vi "Pneumatic Control Loop.vi"(11 "Cluster in":T1) -> ()   [LabVIEW 2015]
uses:
  Support Code/Solenoid Control Loop.ctl
  Support Code/Pneumatics Command.ctl
  Support Code/Pneumatics Position.ctl
  <vilib>/Rock Robotics/WPI/Solenoid/WPI_SolenoidDevRef.ctl
  <vilib>/Rock Robotics/WPI/Solenoid/WPI_SolenoidChannel.ctl
  <vilib>/Rock Robotics/WPI/Solenoid/WPI_SolenoidValue.ctl
  <vilib>/Rock Robotics/WPI/Solenoid/WPI_SolenoidSetEnum.vi
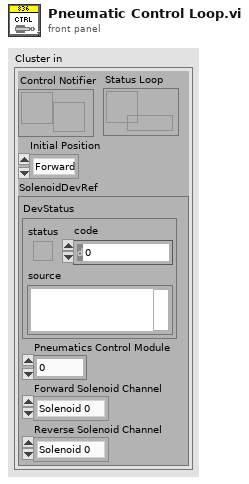
[diagram p1: front panel]
types:
  T1 = typedef "Solenoid Control Loop.ctl" = cluster{"Control Notifier":refnum<notifier>, "Initial Position":T2, "SolenoidDevRef":T3, "Status Loop":refnum<k33>}
  T2 = typedef "Pneumatics Position.ctl" = enum16{"Forward", "Reverse"}
  T3 = typedef "WPI_SolenoidDevRef.ctl" = cluster{"DevStatus":errorcluster, "Pneumatics Control Module":u8, "Forward Solenoid Channel":T4, "Reverse Solenoid Channel":T4}
  T4 = typedef "WPI_SolenoidChannel.ctl" = enum8{"Solenoid 0", "Solenoid 1", "Solenoid 2", "Solenoid 3", "Solenoid 4", "Solenoid 5", "Solenoid 6", "Solenoid 7", "Invalid"}
  T5 = typedef "Pneumatics Command.ctl" = enum16{"Nothing", "Forward", "Reverse", "Toggle"}
  T6 = typedef "WPI_SolenoidValue.ctl" = enum16{"Off", "On", "Forward", "Reverse"}
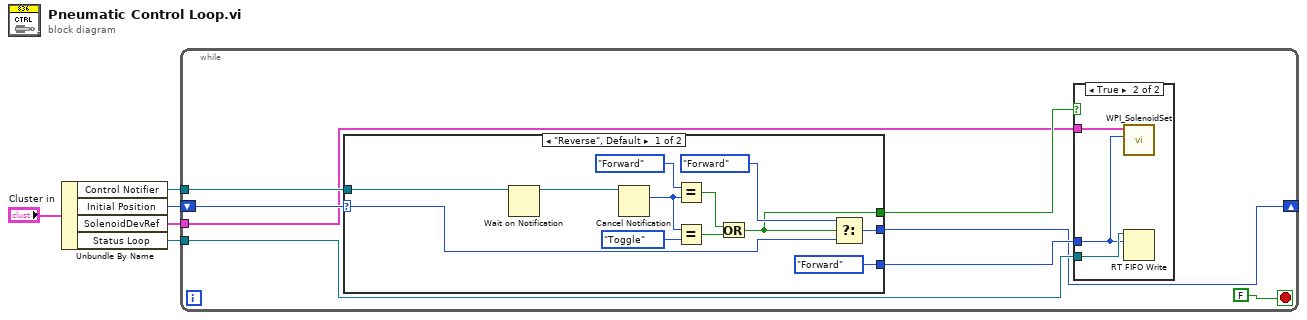
[diagram p0: block diagram]
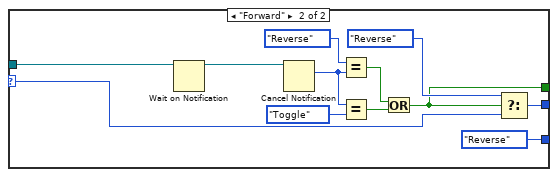
[diagram p3: hidden frame]
diagram:
  n1 = Unbundle By Name("Cluster in") -> ("Control Notifier"=w2:refnum<notifier>, "Initial Position"=w3:T2, "SolenoidDevRef"=w4:T3, "Status Loop"=w5:refnum<k33>)
  n2 = while {
    tunnel: w2 -> [w11]
    shift-right: [w6] -> _
    shift-left: w3 -> [w12]
    tunnel: w4 -> [w8]
    tunnel: w5 -> [w7]
    stop <- FALSE stop-if-true
    n3 = case shown="\"Reverse\", Default" w12 {
      selector: w12 -> [w26 w38]
      tunnel: w11 -> [w28 w40]
      tunnel: [w25 w37] -> w6
      tunnel: [w19 w31] -> w10
      tunnel: [WPI_SolenoidValue."Forward" ("Value") WPI_SolenoidValue."Reverse" ("Value")] -> w9
      frame "Reverse", Default {
        n4 = Wait on Notification(notifier=w28) -> (notifier out=w18:refnum<notifier>)  [unwired: 3 in, 3 out]
        n5 = Cancel Notification(0:w18) -> (9:w17:T5)  [unwired: 1 in, 2 out]
        n6 = Equal?(x=Pneumatics_Command."Forward" ("y"), y=w17) -> (x = y?=w20:bool)
        n7 = Equal?(x=w17, y=Pneumatics_Command."Toggle") -> (x = y?=w21:bool)
        n8 = Or(x=w20, y=w21) -> (x .or. y?=w19:bool)
        n9 = Select(t=Pneumatics_Position."Forward", s=w19, f=w26) -> (s? t:f=w25:T2)
      }
      frame "Forward" {
        n10 = Wait on Notification(notifier=w40) -> (notifier out=w30:refnum<notifier>)  [unwired: 3 in, 3 out]
        n11 = Cancel Notification(0:w30) -> (9:w29:T5)  [unwired: 1 in, 2 out]
        n12 = Equal?(x=Pneumatics_Command."Reverse" ("y"), y=w29) -> (x = y?=w32:bool)
        n13 = Equal?(x=w29, y=Pneumatics_Command."Toggle") -> (x = y?=w33:bool)
        n14 = Or(x=w32, y=w33) -> (x .or. y?=w31:bool)
        n15 = Select(t=Pneumatics_Position."Reverse", s=w31, f=w38) -> (s? t:f=w37:T2)
      }
    }
    n16 = case shown="True" w10 {
      tunnel: w9 -> [_ w14]
      tunnel: w8 -> [_ w16]
      tunnel: w7 -> [_ w15]
      frame False {
      }
      frame True {
        n17 = call-poly <vilib>:"WPI_SolenoidSet.vi"("Value"=w14, "SolenoidDevRef"=w16) -> ()  [unwired: 8 in, 2 out]
        n18 = RT FIFO Write(0:w15, 1:w14) -> ()  [unwired: 3 in, 4 out]
      }
    }
  }
